vi "Log Data.vi"(8 "error in (no error)":errorcluster, 11 "Bioreactor in":refnum<class "Bioreactor.lvclass">) -> (0 "error out":errorcluster, 3 "Bioreactor out":refnum<class "Bioreactor.lvclass">)   [LabVIEW 2012, in "Bioreactor Actor.lvlib" / "Bioreactor.lvclass"]
uses:
  Bioreactor.lvclass
  Bioreactor.lvclass/Bioreactor.ctl
  Read TDMS.vi
  Read DVR.vi
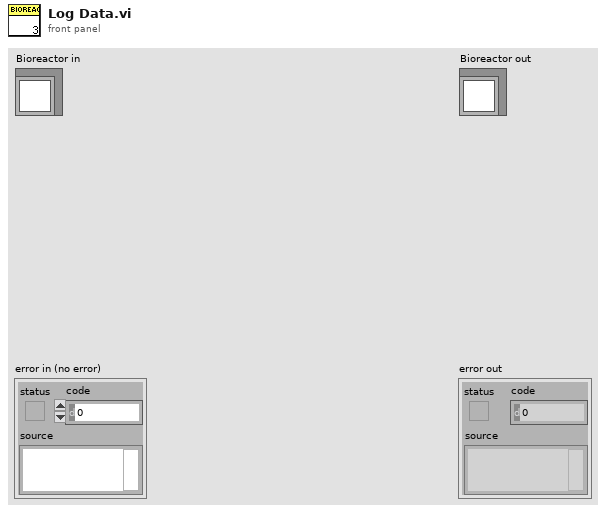
[diagram p1: front panel]
types:
  T1 = cluster{"Name":string, "Value":dbl, "Setpoint":dbl, "Output":dbl}[]
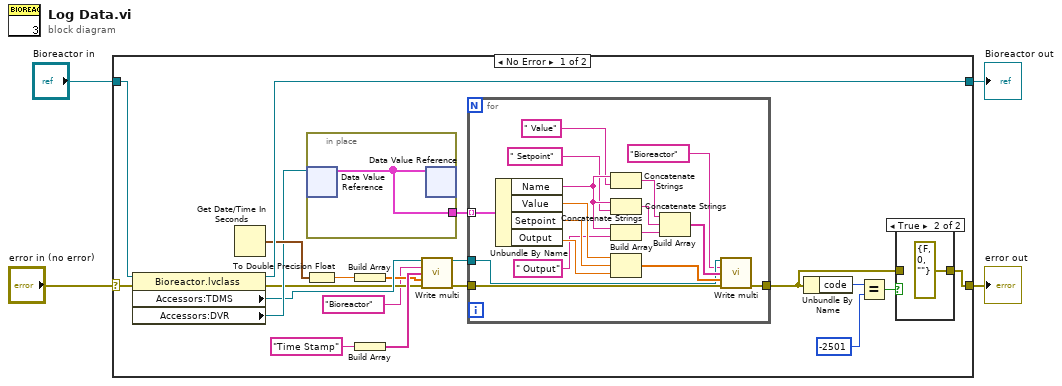
[diagram p0: block diagram]
diagram:
  n1 = case shown="No Error" "error in (no error)" {
    selector: "error in (no error)" -> [w23 w46]
    tunnel: [w21 w46] -> w3
    tunnel: [w22 w45] -> w1
    tunnel: "Bioreactor in" -> [w24 w45]
    frame No Error {
      n2 = property class="Bioreactor.lvclass"(reference=w24, error in=w23) -> (reference out=w22:refnum<class "Bioreactor.lvclass">, error out=w12:errorcluster, "Accessors:TDMS"=w17:refnum<k34>, "Accessors:DVR"=w18:refnum<data-value>)
      n3 = Get Date/Time In Seconds() -> (seconds since 1Jan1904=w20:timestamp)
      n4 = in-place {
        in-place-border: [w44] -> w19
        n5 = in-place-dvr #1(w18) -> (w44:T1)  [unwired: 1 out]
        n6 = in-place-dvr #1(w44) -> ()  [unwired: 2 out]
      }
      n7 = To Double Precision Float(number=w20) -> (double precision float=w14:dbl)
      n8 = Build Array(w14) -> (w13:dbl[])
      n9 = Build Array("Time Stamp" ("Channel")) -> (w15:string[])
      n10 = call "Write multi.vi"("tdms file in"=w17, "group"="Bioreactor", "Channel"=w15, "Data"=w13, "error in (no error)"=w12) -> ("tdms file out"=w10:refnum<k34>, "error out"=w11:errorcluster)  [unwired: 7 in, 2 out]
      n11 = for {
        tunnel: w19 -> [w43] mode=indexing
        tunnel: w11 -> [w30]
        tunnel: [w29] -> w5
        tunnel: w10 -> [w28]
        n12 = Unbundle By Name(w43) -> ("Name"=w39:string, "Value"=w40:dbl, "Setpoint"=w41:dbl, "Output"=w42:dbl)
        n13 = Concatenate Strings(w39, " Value" ("string")) -> (w35:string)
        n14 = Concatenate Strings(w39, " Setpoint" ("string")) -> (w34:string)
        n15 = Concatenate Strings(w39, " Output" ("string")) -> (w33:string)
        n16 = Build Array(w40, w41, w42) -> (w31:dbl[])
        n17 = Build Array(w35, w34, w33) -> (w32:string[])
        n18 = call "Write multi.vi"("tdms file in"=w28, "group"="Bioreactor", "Channel"=w32, "Data"=w31, "error in (no error)"=w30) -> ("error out"=w29:errorcluster)  [unwired: 7 in, 3 out]
      }
      n19 = Unbundle By Name(w5) -> ("code"=w8:i32)
      n20 = Equal?(x=w8, y=-2501) -> (x = y?=w6:bool)
      n21 = case shown="True" w6 {
        tunnel: w5 -> [w25 _]
        tunnel: [w25 errorcluster {"status"=FALSE, "code"=0, "source"=""} ("error constant")] -> w21
        frame False {
        }
        frame True {
        }
      }
    }
    frame Error {
    }
  }
  "error out" <- w3
  "Bioreactor out" <- w1
